vi "camera_closer.vi"(0 "input cluster":T3) -> ()   [LabVIEW 2015]
uses:
  <vilib>/vision/Avi1.llb/AviRefnum.ctl
  <vilib>/userdefined/High Color/IMAQdx.ctl
  <vilib>/vision/driver/NI_Vision_Acquisition_Software.lvlib
panel:
  out "AVI error out":errorcluster
  out "IMAQdx error out":errorcluster
  out "IMAQ error out":errorcluster
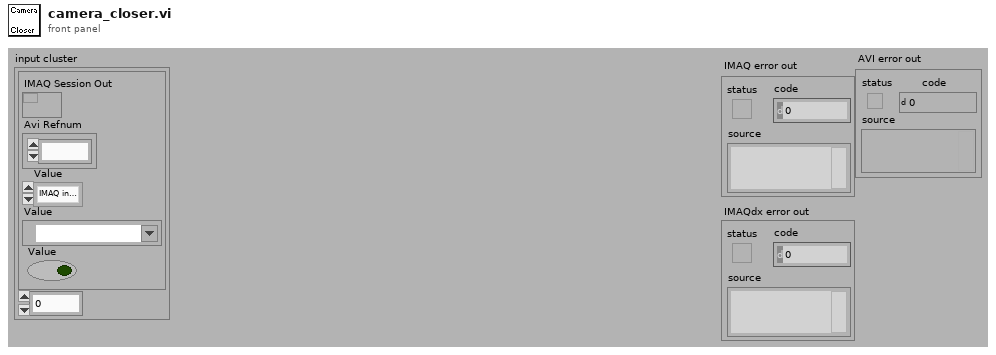
[diagram p1: front panel]
types:
  T1 = typedef "AviRefnum.ctl" = refnum<k1>
  T2 = typedef "IMAQdx.ctl" = refnum<k21>
  T3 = cluster{cluster{"IMAQ Session Out":refnum<k11>, "Avi Refnum":T1, "Value":enum32{"IMAQ interface", "IMAQdx interface", "AVI file"}, "Value":T2, "Value":bool}, i32}
  T4 = cluster{"IMAQ Session Out":refnum<k11>, "Avi Refnum":T1, "Value":enum32{"IMAQ interface", "IMAQdx interface", "AVI file"}, "Value":T2, "Value":bool}
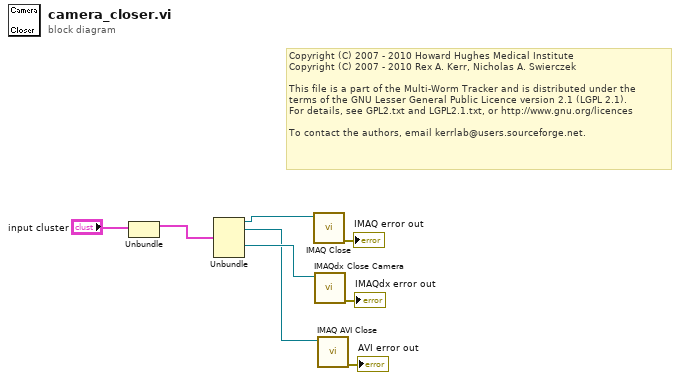
[diagram p0: block diagram]
diagram:
  # "Copyright (C) 2007 - 2010 Howard Hughes Medical Institute\nCopyright (C) 2007 - 2010 Rex A. Kerr, Nicholas A. Swierczek\n \nThis file is a part of the Multi-Worm Tracker and is distributed under the\nterms of the GNU Lesser General Public Licence version 2.1 (LGPL 2.1).\nFor details, see GPL2.txt and LGPL2.1.txt, or http://www.gnu.org/licences\n \nTo contact the authors, email kerrlab@users.sourceforge.net."
  n1 = Unbundle("input cluster") -> (w8:T4)  [unwired: 1 out]
  n2 = Unbundle(w8) -> ("IMAQ Session Out"=w7:refnum<k11>, "Avi Refnum"=w2:T1, "Value"=w3:T2)  [unwired: 2 out]
  n3 = call <vilib>:"IMAQ Close.vi"("IMAQ Session In"=w7) -> ("error out"=→"IMAQ error out":errorcluster)  [unwired: 10 in]
  n4 = call <vilib>:"IMAQdx Close Camera.vi"("Session In"=w3) -> ("error out"=→"IMAQdx error out":errorcluster)  [unwired: 10 in]
  n5 = call "IMAQ AVI Close"("Avi Refnum"=w2) -> ("error out"=→"AVI error out":errorcluster)  [unwired: 10 in]
